vi "KH_EthernetIP_Globals.vi"() -> ()   [LabVIEW 2017]
uses:
  KH EthernetIPConfig 17.14/KH EthernetIPConfig TDef Config.ctl
  KH EthernetIPConfig 17.14/KH EthernetIPConfig TypeDefs ModuleTyp.ctl
panel:
  in  "OtoT NetworkConnID":u32[](array[numeric]) format="%.0x"
  in  "TtoO NetworkConnID":u32[](array[numeric]) format="%.0x"
  in  "Config":T1[](array[typedef])
  out "Server EthernetIP":bool
  in  "EthernetIP Simulation":bool=TRUE
  out "EthernetIP Global Stop":bool
  in  "EthernetIP_tab":enum32{"Connection"}(tab)
  in  "Connection Feedback":T3(array[cluster]) {"ConnectionSerialNumber" format="%.0x"; "OriginatorSerialNumber" format="%.0x"; "OtoT NetworkConnID" format="%.0x"; "TtoO NetworkConnID" format="%.0x"}
  in  "ConnectionData":T4(array[cluster]) {"TtoO ConnPointSegmValue" format="%.0x"; "TtoO ConnPointSegment" format="%.0x"; "OtoT ConnPointSegmValue" format="%.0x"; "OtoT ConnPointSegment" format="%.0x"; "Instance ID" format="%.0x"; "Instance ID Descriptor" format="%.0x"; "Class ID" format="%.0x"; "Class ID Descriptor" format="%.0x"; "TtoO NetworkConnParam" format="%.0x"; "OtoT NetworkConnParam" format="%.0x"}
  out "TCP Connection IDs":refnum<k5>[](array[refnum])
  out "SessionHandles":u32[](array[numeric]) format="%.0x"
  in  "remote port":u16=44818
  in  "local port UDP":u16=61556
  in  "timeout":i32=61556
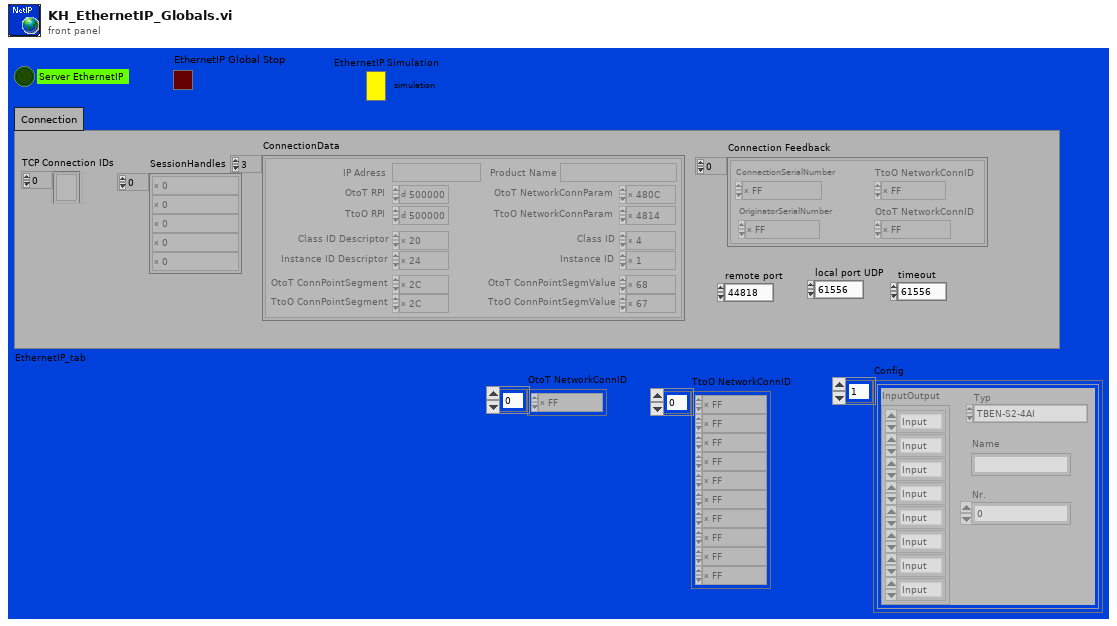
[diagram p1: front panel]
types:
  T1 = typedef "KH EthernetIPConfig TDef Config.ctl" = cluster{"Typ":T2, "Name":string, "Nr.":i32, "InputOutput":enum16{"Input", "Output"}[]}
  T2 = typedef "KH EthernetIPConfig TypeDefs ModuleTyp.ctl" = enum16{"TBEN-S2-4AI", "TBEN-S1-8DXP", "TBEN-S2-2RFID-4DXP", "TBEN-S2-4AO", "TBEN-S2-4IOL"}
  T3 = cluster{"TtoO NetworkConnID":u32, "OtoT NetworkConnID":u32, "OriginatorSerialNumber":u32, "ConnectionSerialNumber":u16}[]
  T4 = cluster{"OtoT RPI":u32, "OtoT NetworkConnParam":u16, "TtoO RPI":u32, "TtoO NetworkConnParam":u16, "Class ID Descriptor":u8, "Class ID":u8, "Instance ID Descriptor":u8, "Instance ID":u8, "OtoT ConnPointSegment":u8, "OtoT ConnPointSegmValue":u8, "TtoO ConnPointSegment":u8, "TtoO ConnPointSegmValue":u8, "IP Adress":string, "Product Name":string}[]
diagram:
